vi "StopSync.vi"(8 "error in (no error)":errorcluster, 11 "NiPxi6683H in":refnum<class "NiPxi6683H.lvclass">) -> (0 "error out":errorcluster, 3 "NiPxi6683H out":refnum<class "NiPxi6683H.lvclass">)   [LabVIEW 2014, in "SyncPlugins.lvlib" / "NiPxi6683H.lvclass"]
uses:
  NiPxi6683H.lvclass
  NiPxi6683H.lvclass/NiPxi6683H.ctl
  NiPxi6682/NiPxi6682.lvclass/NiPxi6682.ctl
  SyncPluginBase/SyncPluginBase.lvclass/SyncPluginBase.ctl
  Accessors/Read Triggers.vi
  Accessors/Read Clocks.vi
  NiPxi6682/Accessors/Read NiSyncHandle.vi
  SyncPluginBase/Accessors/Write Initiated.vi
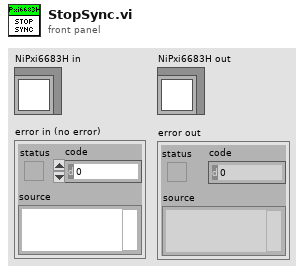
[diagram p1: front panel]
types:
  T1 = typedef "SyncPlugins.lvlib/PXI_MultiTrig.lvclass/clTrigger.ctl" = cluster{"Name":string, "DestTerm":string, "SrcTerm":string, "SyncClk":string, "Edge":i32, "Invert?":i32, "Initiated":bool, "Type":string, "TrigTime":bool}
  T2 = typedef "SyncPlugins.lvlib/PXI_MultiTrig.lvclass/clClocks.ctl" = cluster{"Name":string, "RefClk":string, "ClkTerminal":string, "Frequency":dbl, "DutyCycle":dbl, "ClkType":string, "Initiated":bool, "TrigTime":bool}
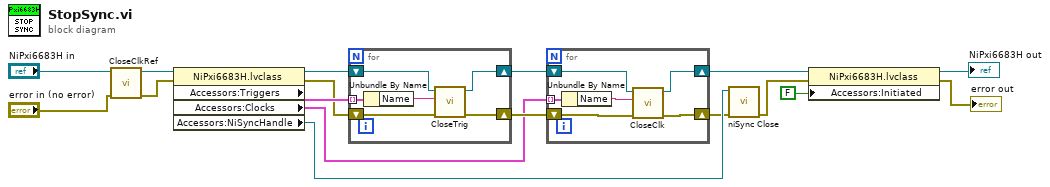
[diagram p0: block diagram]
diagram:
  n1 = call "CloseClkRef.vi"("error in (no error)"="error in (no error)", "NiPxi6683H in"="NiPxi6683H in") -> ("error out"=w15:errorcluster, "NiPxi6683H out"=w14:refnum<class "NiPxi6683H.lvclass">)  [unwired: 8 in]
  n2 = property class="NiPxi6683H.lvclass"(reference=w14, error in=w15) -> (reference out=w13:refnum<class "NiPxi6683H.lvclass">, error out=w11:errorcluster, "Accessors:Triggers"=w12:T1[], "Accessors:Clocks"=w5:T2[], "Accessors:NiSyncHandle"=w3:refnum<k15>)
  n3 = for {
    shift-right: [w22] -> w7
    shift-left: w11 -> [w23]
    shift-right: [w20] -> w6
    shift-left: w13 -> [w21]
    tunnel: w12 -> [w18] mode=indexing
    n4 = Unbundle By Name(w18) -> ("Name"=w19:string)
    n5 = call-dynamic "CloseTrig.vi"("error in (no error)"=w23, "ClkName"=w19, "NiPxi6683H in"=w21) -> ("error out"=w22:errorcluster, "NiPxi6683H out"=w20:refnum<class "NiPxi6683H.lvclass">)  [unwired: 7 in]
  }
  n6 = for {
    shift-right: [w28] -> w2
    shift-left: w7 -> [w29]
    shift-right: [w26] -> w4
    shift-left: w6 -> [w27]
    tunnel: w5 -> [w24] mode=indexing
    n7 = Unbundle By Name(w24) -> ("Name"=w25:string)
    n8 = call-dynamic "CloseClk.vi"("error in (no error)"=w29, "ClkName"=w25, "NiPxi6683H in"=w27) -> ("error out"=w28:errorcluster, "NiPxi6683H out"=w26:refnum<class "NiPxi6683H.lvclass">)  [unwired: 7 in]
  }
  n9 = call <instrlib>:"niSync Close.vi"("error in (no error)"=w2, "instrument handle"=w3) -> ("error out"=w1:errorcluster)  [unwired: 9 in]
  n10 = property class="NiPxi6683H.lvclass"(reference=w4, error in=w1, "Accessors:Initiated"=FALSE ("Initiated")) -> (reference out=→"NiPxi6683H out":refnum<class "NiPxi6683H.lvclass">, error out=→"error out":errorcluster)
